vi "DownloadSpriteImages.vi"(8 "error in (no error)":errorcluster, 10 "Sprites in":refnum<class "RT_Sprite.lvclass">[](array[class]), 11 "Engine in":refnum<class "Engine.lvclass">) -> (0 "error out":errorcluster, 3 "Engine out":refnum<class "Engine.lvclass">)   [LabVIEW 2019, in "RT_Game.lvlib" / "Engine.lvclass"]
uses:
  Engine.lvclass
  RT_Sprite/RT_Sprite.lvclass
  Engine.lvclass/Engine.ctl
  RT_Sprite/RT_Sprite.lvclass/RT_Sprite.ctl
  RT_Sprite/Read Picture.vi
  <vilib>/Utility/error.llb/Error Cluster From Error Code.vi
  <vilib>/rvi/errors/niLvFpgaAdjustHostInterfaceError.vi
  <vilib>/rvi/interface/nirviReadWriteControl/nirviReadWriteControl.xnode
  FPGA_Interface.ctl
  FPGA Bitfiles/myriogameconsole_FPGATarget_Main_ntsPRcBZGxk.lvbitx
  <vilib>/rvi/interface/nirviMethod/nirviMethod.xnode
  <vilib>/FPGAPlugInAG/myRIO-1900/niLvFpga_WriteFifo_myRIO-1900.vi
  <vilib>/rvi/errors/niLvFpgaMergeErrorWithErrorCode.vi
  NiFpgaLv.dll
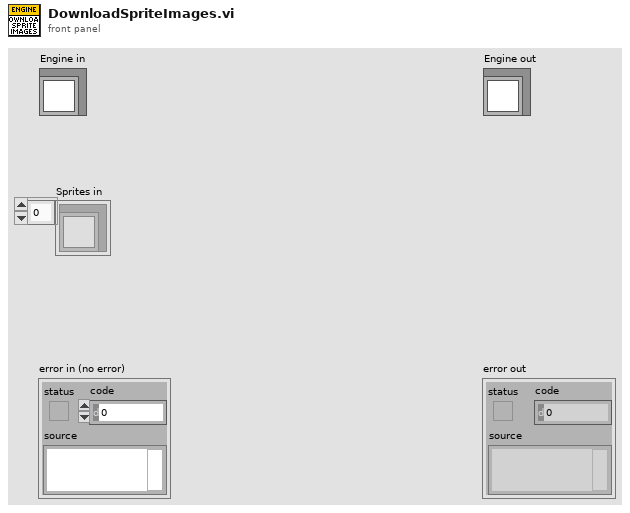
[diagram p1: front panel]
types:
  T1 = typedef "FPGA_Interface.ctl" = refnum<k20>
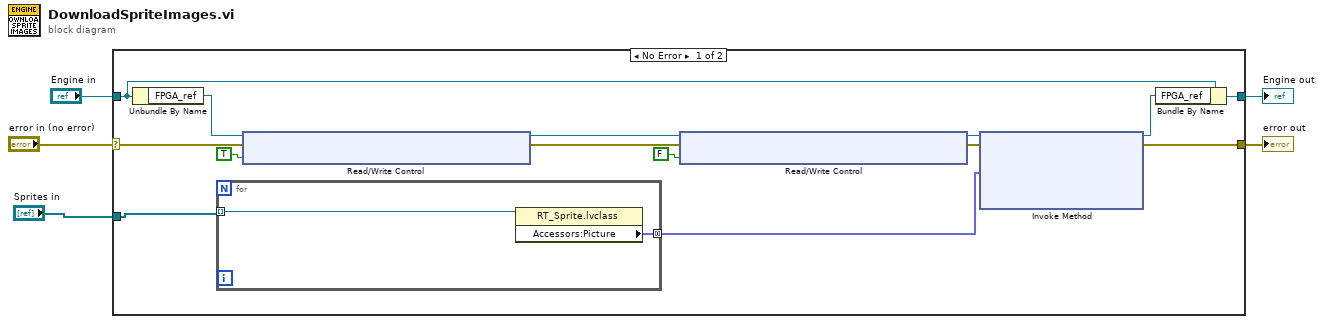
[diagram p0: block diagram]
diagram:
  n1 = case shown="No Error" "error in (no error)" {
    selector: "error in (no error)" -> [w13 w23]
    tunnel: [w12 w23] -> w4
    tunnel: [w11 w22] -> w2
    tunnel: "Engine in" -> [w9 w22]
    tunnel: "Sprites in" -> [w6 _]
    frame No Error {
      n2 = Unbundle By Name(w9) -> ("FPGA_ref"=w8:T1)
      n3 = for {
        tunnel: w6 -> [w21] mode=indexing
        tunnel: [w20] -> w14 mode=concatenating
        n4 = property class="RT_Sprite.lvclass"(reference=w21) -> ("Accessors:Picture"=w20:fxp<+,3,3>[])  [unwired: 1 in, 2 out]
      }
      n5 = xnode "Read/Write Control"("FPGA VI Reference In"=w8, "error in"=w13, "Spritesetbuffer_ResetAddress"=TRUE ("Spritebuffer_ResetAddress")) -> ("FPGA VI Reference Out"=w7:T1, "error out"=w15:errorcluster)
      n6 = xnode "Read/Write Control"("FPGA VI Reference In"=w7, "error in"=w15, "Spritesetbuffer_ResetAddress"=FALSE ("Spritebuffer_ResetAddress")) -> ("FPGA VI Reference Out"=w18:T1, "error out"=w16:errorcluster)
      n7 = xnode "Invoke Method"("FPGA VI Reference In"=w18, "error in"=w16, "Data"=w14) -> ("FPGA VI Reference Out"=w10:T1, "error out"=w12:errorcluster)  [unwired: 1 in, 1 out]
      n8 = Bundle By Name(cluster=w9, "FPGA_ref"=w10) -> (w11:refnum<class "Engine.lvclass">)
    }
    frame Error {
    }
  }
  "error out" <- w4
  "Engine out" <- w2
